vi "ConvertStringTemperatureToNumeric.vi"(11 "Temperature":string) -> (2 "Connected?":bool, 3 "Temperature (C)":dbl)   [LabVIEW 2012, in "Omega-CSi32.lvlib"]
uses:
  Omega-CSi32.lvlib
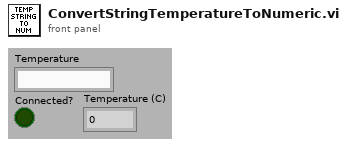
[diagram p1: front panel]
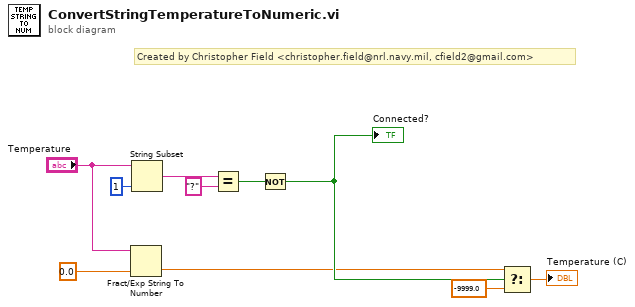
[diagram p0: block diagram]
diagram:
  # "Created by Christopher Field <christopher.field@nrl.navy.mil, cfield2@gmail.com>"
  n1 = Fract/Exp String To Number(string="Temperature", default (0 dbl)=0.0 ("default (0 DBL)")) -> (number=w4:dbl)  [unwired: 2 in, 1 out]
  n2 = String Subset(string="Temperature", length (rest)=1 ("length (rest)")) -> (substring=w9:string)  [unwired: 1 in]
  n3 = Equal?(x=w9, y="?") -> (x = y?=w7:bool)
  n4 = Not(x=w7) -> (.not. x?=w6:bool)
  "Connected?" <- w6
  n5 = Select(t=w4, s=w6, f=-9999.0) -> (s? t:f=→"Temperature (C)":dbl)
